vi "untitled.vi"() -> ()   [LabVIEW 2023]
panel:
  in  "stop":bool
  out "Diode 2":bool
  out "Diode 1":bool
  out "Numeric":dbl
  out "Waveform Graph 2":waveform(dbl)[](graph)
  out "Waveform Graph":dbl[][](graph)
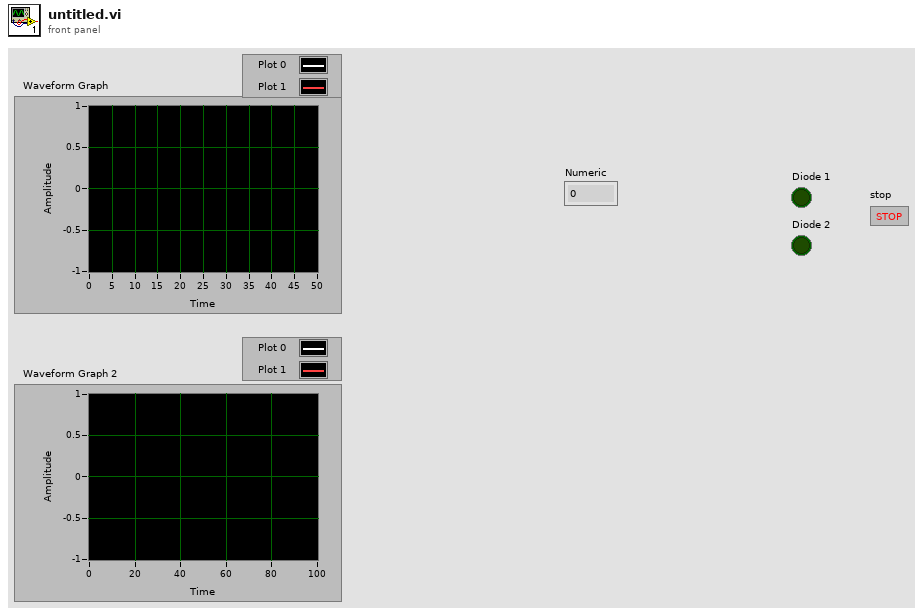
[diagram p1: front panel]
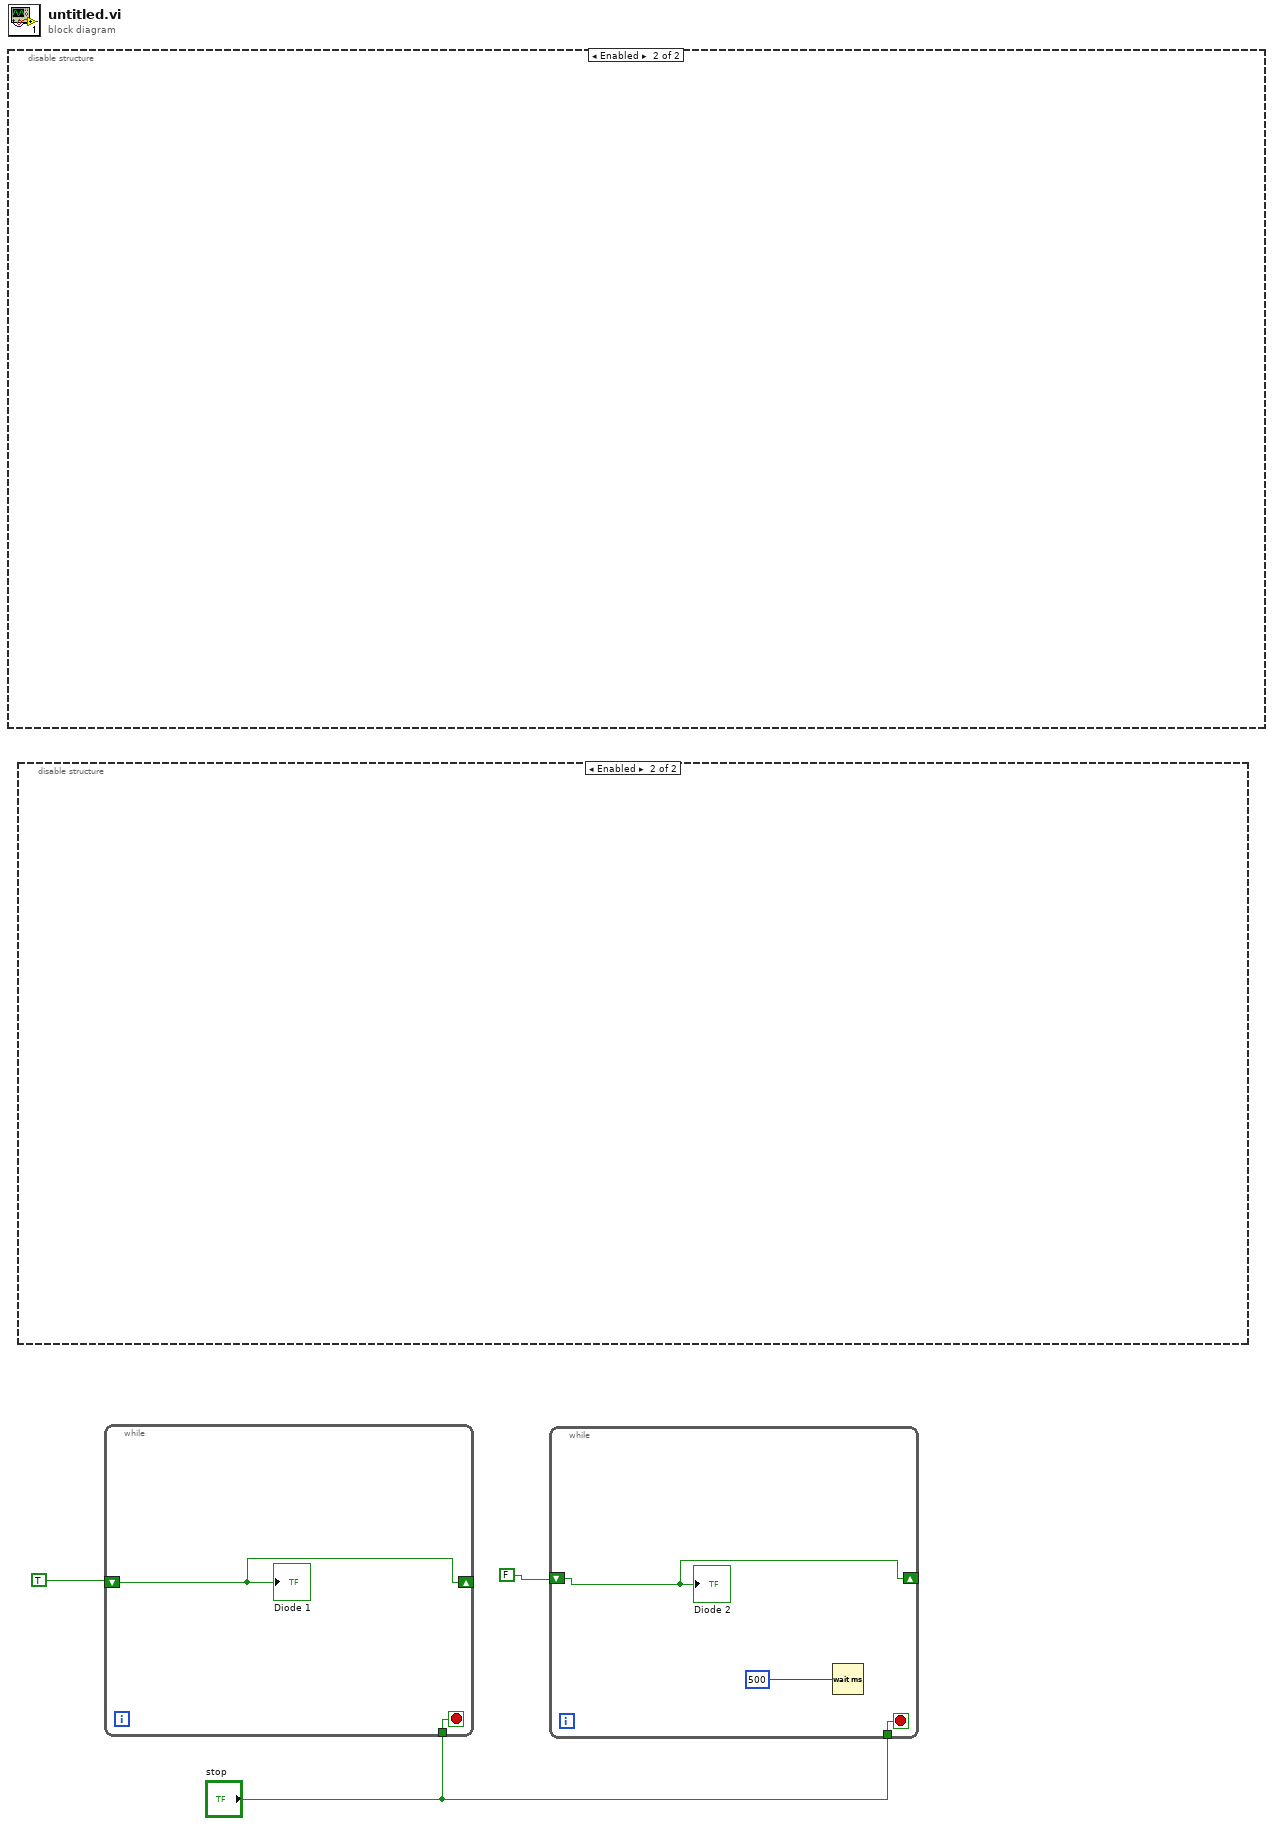
[diagram p0: block diagram]
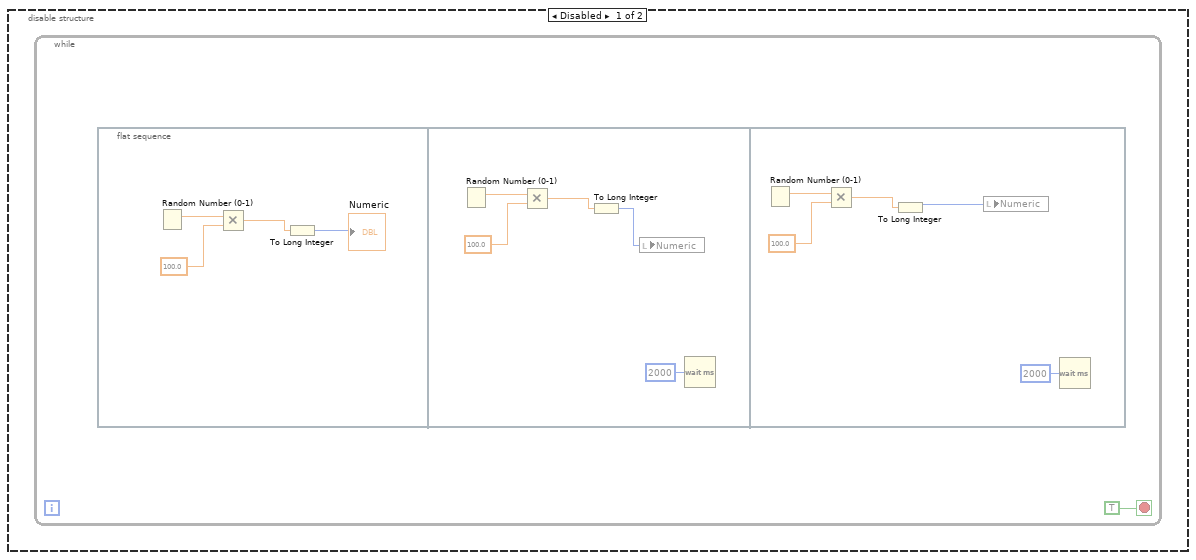
[diagram p2: hidden frame]
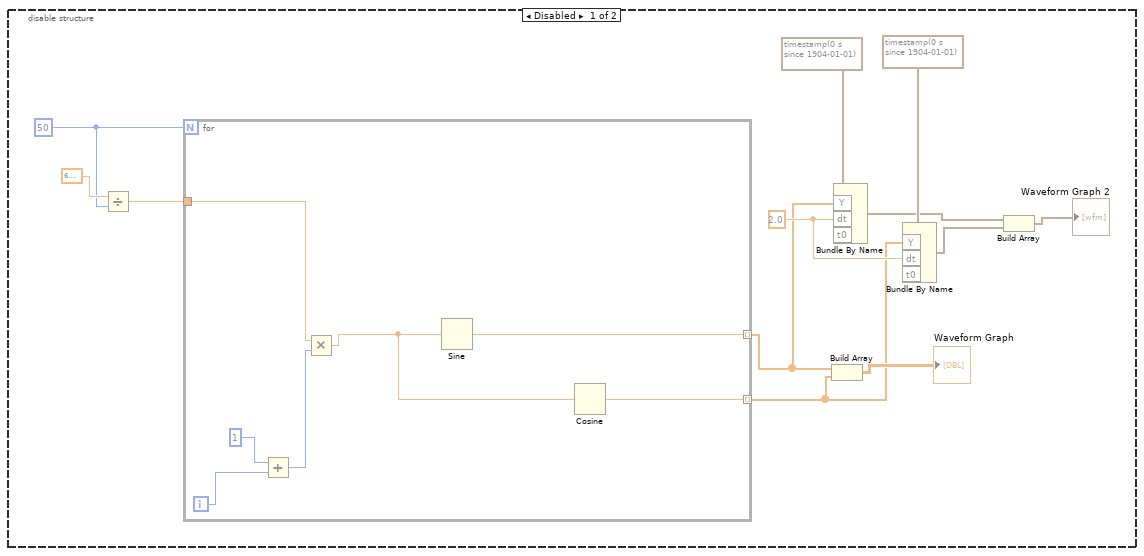
[diagram p3: hidden frame]
diagram:
  n1 = disable-structure shown="Enabled" {
    frame Disabled {
      w9 = 2.0 ("dt")
      w13 = 50
      n2 = Divide(x=6.283185307179586, y=w13) -> (x/y=w15:dbl)
      n3 = for {
        N: w13 -> [_]
        tunnel: w15 -> [w20]
        tunnel: [w18] -> w8 mode=indexing
        tunnel: [w16] -> w7 mode=indexing
        i -> [w22]
        n4 = Add(x=1, y=w22) -> (x+y=w19:i32)
        n5 = Multiply(x=w20, y=w19) -> (x*y=w17:dbl)
        n6 = Sine(x=w17) -> (sin(x)=w18:dbl)
        n7 = Cosine(x=w17) -> (cos(x)=w16:dbl)
      }
      n8 = Build Array(w8, w7) -> (→"Waveform Graph":dbl[][])
      n9 = Bundle By Name("Y"=w8, "dt"=w9, "t0"=timestamp(0 s since 1904-01-01)) -> (w6:waveform(dbl))  [unwired: 1 in]
      n10 = Bundle By Name("Y"=w7, "dt"=w9, "t0"=timestamp(0 s since 1904-01-01)) -> (w5:waveform(dbl))  [unwired: 1 in]
      n11 = Build Array(w6, w5) -> (→"Waveform Graph 2":waveform(dbl)[])
    }
    frame Enabled {
    }
  }
  n12 = disable-structure shown="Enabled" {
    frame Disabled {
      n13 = while {
        stop <- TRUE stop-if-true
        n14 = flat-sequence {
          frame #0 {
            n15 = Random Number (0-1)() -> (number: 0 to 1=w27:dbl)
            n16 = Multiply(x=w27, y=100.0) -> (x*y=w24:dbl)
            n17 = To Long Integer(number=w24) -> (32bit integer=→"Numeric":i32)
          }
          frame #1 {
            n18 = Random Number (0-1)() -> (number: 0 to 1=w29:dbl)
            n19 = Multiply(x=w29, y=100.0) -> (x*y=w31:dbl)
            n20 = To Long Integer(number=w31) -> (32bit integer=w28:i32)
            n21 = local write "Numeric"(w28) -> ()
            n22 = Wait (ms)(milliseconds to wait=u32 2000) -> ()  [unwired: 1 out]
          }
          frame #2 {
            n23 = Random Number (0-1)() -> (number: 0 to 1=w37:dbl)
            n24 = Multiply(x=w37, y=100.0) -> (x*y=w35:dbl)
            n25 = To Long Integer(number=w35) -> (32bit integer=w34:i32)
            n26 = local write "Numeric"(w34) -> ()
            n27 = Wait (ms)(milliseconds to wait=u32 2000) -> ()  [unwired: 1 out]
          }
        }
      }
    }
    frame Enabled {
    }
  }
  n28 = while {
    shift-right: [w38] -> _
    shift-left: TRUE -> [w38]
    tunnel: "stop" -> [w39]
    stop <- w39 stop-if-true
    "Diode 1" <- w38
  }
  n29 = while {
    shift-right: [w40] -> _
    shift-left: FALSE -> [w40]
    tunnel: "stop" -> [w42]
    stop <- w42 stop-if-true
    n30 = Wait (ms)(milliseconds to wait=u32 500) -> ()  [unwired: 1 out]
    "Diode 2" <- w40
  }
